vi "DetermineCompressionInfo.vi"(8 "error in (no error)":errorcluster, 10 "connections (ID)":string, 11 "Variant In":variant) -> (0 "error out":errorcluster, 1 "non compressed":bool, 2 "compressed":bool, 3 "Variant Out":variant)   [LabVIEW 2011]
uses:
  connectiondata_typdef.ctl
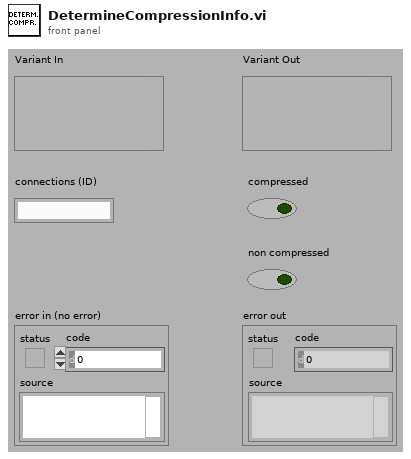
[diagram p1: front panel]
types:
  T1 = typedef "connectiondata_typdef.ctl" = cluster{"connection ID":refnum<k5>, "local":bool, "spawn":bool, "variable(s)":string}
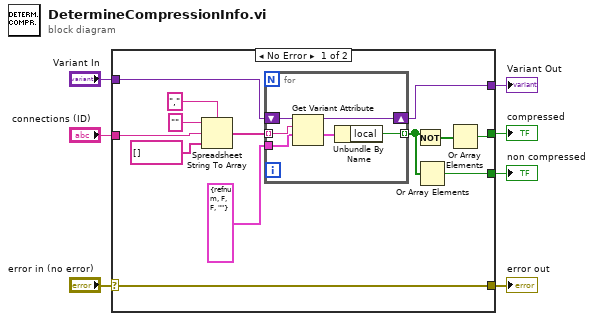
[diagram p0: block diagram]
diagram:
  n1 = case shown="No Error" "error in (no error)" {
    selector: "error in (no error)" -> [w11 w27]
    tunnel: [w8 _] -> w7
    tunnel: [w20 _] -> w6
    tunnel: "connections (ID)" -> [w15 _]
    tunnel: [w13 w28] -> w4
    tunnel: "Variant In" -> [w12 w28]
    tunnel: [w11 w27] -> w1
    frame No Error {
      n2 = Spreadsheet String To Array(delimiter (Tab)="," ("format string"), format string="", spreadsheet string=w15, array type (2D Dbl)=string[] []) -> (array=w17:string[])
      n3 = for {
        shift-right: [w25] -> w13
        shift-left: w12 -> [w26]
        tunnel: w17 -> [w24] mode=indexing
        tunnel: T1 {"connection ID"=refnum, "local"=FALSE, "spawn"=FALSE, "variable(s)"=""} ("connection data") -> [w23]
        tunnel: [w21] -> w10 mode=indexing
        n4 = Get Variant Attribute(Variant=w26, name=w24, default value (empty Variant)=w23) -> (duplicate Variant=w25:variant, value=w22:T1)  [unwired: 1 in, 2 out]
        n5 = Unbundle By Name(w22) -> ("local"=w21:bool)
      }
      n6 = Not(x=w10) -> (.not. x?=w9:bool[])
      n7 = Or Array Elements(Boolean array=w10) -> (logical OR=w20:bool)
      n8 = Or Array Elements(Boolean array=w9) -> (logical OR=w8:bool)
    }
    frame Error {
    }
  }
  "compressed" <- w7
  "non compressed" <- w6
  "Variant Out" <- w4
  "error out" <- w1
